vi "ADI_IMU_ADIS16470_RefNum Registry Set.vi"(8 "error in (no error)":errorcluster, 10 "refnum name":string="ADIIMURefNum", 11 "ADI IMU DevRef":T1) -> (0 "error out":errorcluster, 3 "ADI IMU DevRef":T1)   [LabVIEW 2017, in "ADIS16470_IMU.lvlib"]
doc: "Sets a reference into a registry so that other VIs can call the reference. After you set a reference, you can call that reference with ADI_IMU_RefNum Registry Get VI."
uses:
  ADIS16470_IMU.lvlib
  ADI_IMU_ADIS16470_IMUDevRef.ctl
  <vilib>/Rock Robotics/SystemInterfaces/spilib/spi_bus.ctl
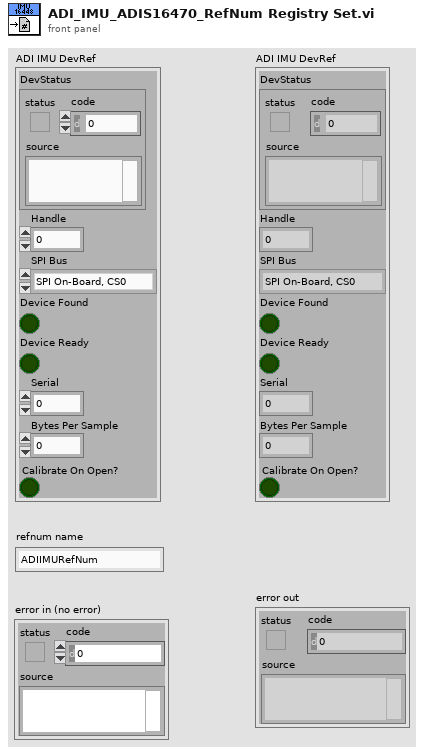
[diagram p1: front panel]
types:
  T1 = typedef "ADIS16470_IMU.lvlib/ADI_IMU_ADIS16470_IMUDevRef.ctl" = cluster{"DevStatus":errorcluster, "Handle":i32, "SPI Bus":T2, "Device Found":bool, "Device Ready":bool, "Serial":u16, "Bytes Per Sample":u16, "Calibrate On Open?":bool}
  T2 = typedef "spi_bus.ctl" = enum16{"SPI On-Board, CS0", "SPI On-Board, CS1", "SPI On-Board, CS2", "SPI On-Board, CS3", "SPI MXP", "Invalid"}
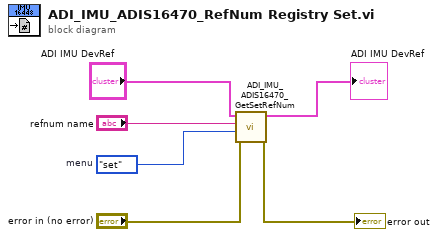
[diagram p0: block diagram]
diagram:
  w4 = enum16{"set", "get", "delete"}."set"  # menu
  n1 = call "ADI_IMU_ADIS16470_GetSetRefNum.vi"("error in (no error)"="error in (no error)", "menu"=w4, "refnum name"="refnum name", "ADI IMU DevRef Set"="ADI IMU DevRef") -> ("error out"=→"error out":errorcluster, "ADI IMU DevRef Get"=→"ADI IMU DevRef":T1)  [unwired: 6 in]
